vi "Main.vi"   [LabVIEW 2015]
doc: "The myRIO Project template acquires acceleration data from the onboard accelerometer and displays the changes of acceleration values in a waveform chart."
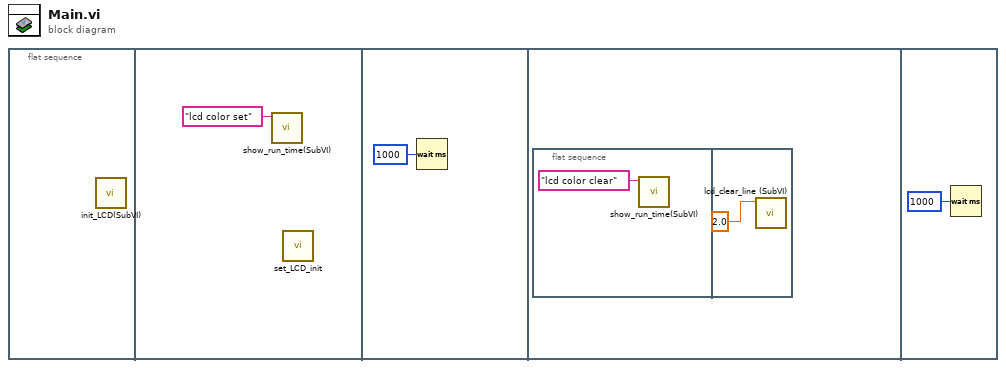
[diagram p0: block diagram]
diagram:
  n1 = flat-sequence {
    frame #0 {
      n2 = call "init_LCD(SubVI).vi"() -> ()  [unwired: 12 in]
    }
    frame #1 {
      n3 = call "show_run_time(SubVI).vi"("String"="lcd color set") -> ()  [unwired: 11 in]
      n4 = call "set_LCD_init.vi"() -> ()  [unwired: 12 in]
    }
    frame #2 {
      n5 = Wait (ms)(milliseconds to wait=u32 1000) -> ()  [unwired: 1 out]
    }
    frame #3 {
      n6 = flat-sequence {
        frame #0 {
          n7 = call "show_run_time(SubVI).vi"("String"="lcd color clear") -> ()  [unwired: 11 in]
        }
        frame #1 {
          n8 = call "lcd_clear_line (SubVI).vi"("Numeric"=2.0) -> ()  [unwired: 11 in]
        }
      }
    }
    frame #4 {
      n9 = Wait (ms)(milliseconds to wait=u32 1000) -> ()  [unwired: 1 out]
    }
  }
